vi "test Compile RaF Channel Data.vi"(8 "error in (no error)":errorcluster, 11 "TestCase in":refnum<class "Routing and Faulting Compile Unit Tests.lvclass">) -> (0 "error out":errorcluster, 3 "TestCase out":refnum<class "Routing and Faulting Compile Unit Tests.lvclass">)   [LabVIEW 2020, in "Routing and Faulting Compile Unit Tests.lvclass"]
uses:
  Routing and Faulting Compile Unit Tests.lvclass
  Shared/Channel States.ctl
  Shared/Routing State.ctl
  Shared/Connection.ctl
  Shared/Compiled.Settings.ctl
  Shared/Communication Configuration.ctl
  Shared/Routing and Faulting Configuration.ctl
  Shared/Routing Channel Configuration.ctl
  Shared/Value-Connections Map.ctl
  Shared/Alias Mapping.ctl
  Shared/Alias Endpoint.ctl
  Shared/Compiled Connection.ctl
  Shared/FIFO Indices.ctl
  Routing and Faulting Compile Unit Tests.lvclass/Routing and Faulting Compile Unit Tests.ctl
  System Explorer/Get Channel Data in By Channel ID (offline).vi
  Scripting/Routing and Faulting Scripting.lvlib
  Shared/Routing and Faulting Shared.lvlib
  System Explorer/Routing and Faulting System Explorer.lvlib
panel:
  in  "Save?":bool
  out "Output Filename":string
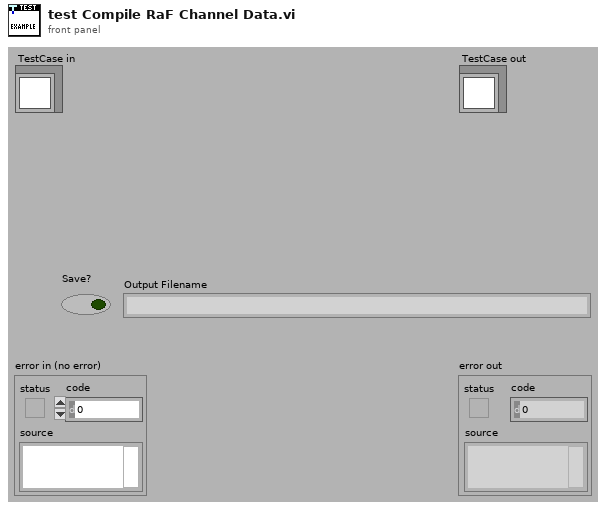
[diagram p1: front panel]
types:
  T1 = typedef "Routing and Faulting Shared.lvlib/Alias Endpoint.ctl" = cluster{"Module Path":string, "Endpoint":string}
  T2 = cluster{"Value-Connections Map.Connection List Array":cluster{"Compiled Connections Indices":i32[]}[]}[]
  T3 = typedef "Routing and Faulting Shared.lvlib/Compiled Connection.ctl" = cluster{"Consumer Queue Index":i32, "Normalized Connection String":string}
  T4 = typedef "Routing and Faulting Shared.lvlib/Communication Configuration.ctl" = cluster{"Consumer Queue Names":string[]}
  T5 = typedef "Routing and Faulting Shared.lvlib/Compiled.Settings.ctl" = cluster{"Custom Device Name":string, "Communication Configuration":T4, "Routing and Faulting Configuration":T6, "Status Channels FIFO Indices":T10}
  T6 = typedef "Routing and Faulting Shared.lvlib/Routing and Faulting Configuration.ctl" = cluster{"Routing Channel Configurations":T7[], "Alias Mappings":T9[], "Compiled Connection Buffer":T3[], "Compiled Initial Connection Indices":i32[]}
  T7 = typedef "Routing and Faulting Shared.lvlib/Routing Channel Configuration.ctl" = cluster{"Channel Name":string, "Initial Value":dbl, "FIFO Index":i32, "Value-Connections Map":T8}
  T8 = typedef "Routing and Faulting Shared.lvlib/Value-Connections Map.ctl" = cluster{"State Value Array":i32[], "Connection List Array":cluster{"Compiled Connections Indices":i32[]}[]}
  T9 = typedef "Routing and Faulting Shared.lvlib/Alias Mapping.ctl" = cluster{"Alias":string, "Endpoint":T1}
  T10 = typedef "Routing and Faulting Shared.lvlib/FIFO Indices.ctl" = cluster{"Status Channel":i32, "Heartbeat Channel":i32}
  T11 = typedef "Routing and Faulting Shared.lvlib/Channel States.ctl" = T12[]
  T12 = typedef "Routing and Faulting Shared.lvlib/Routing State.ctl" = cluster{"Name":string, "Description":string, "Value":i32, "Connection List":T13[]}
  T13 = typedef "Routing and Faulting Shared.lvlib/Connection.ctl" = cluster{"Module":string, "Source":string, "Destination":string}
  T14 = typedef "Custom Device API.lvlib/Custom Device Item Ref.ctl" = u64
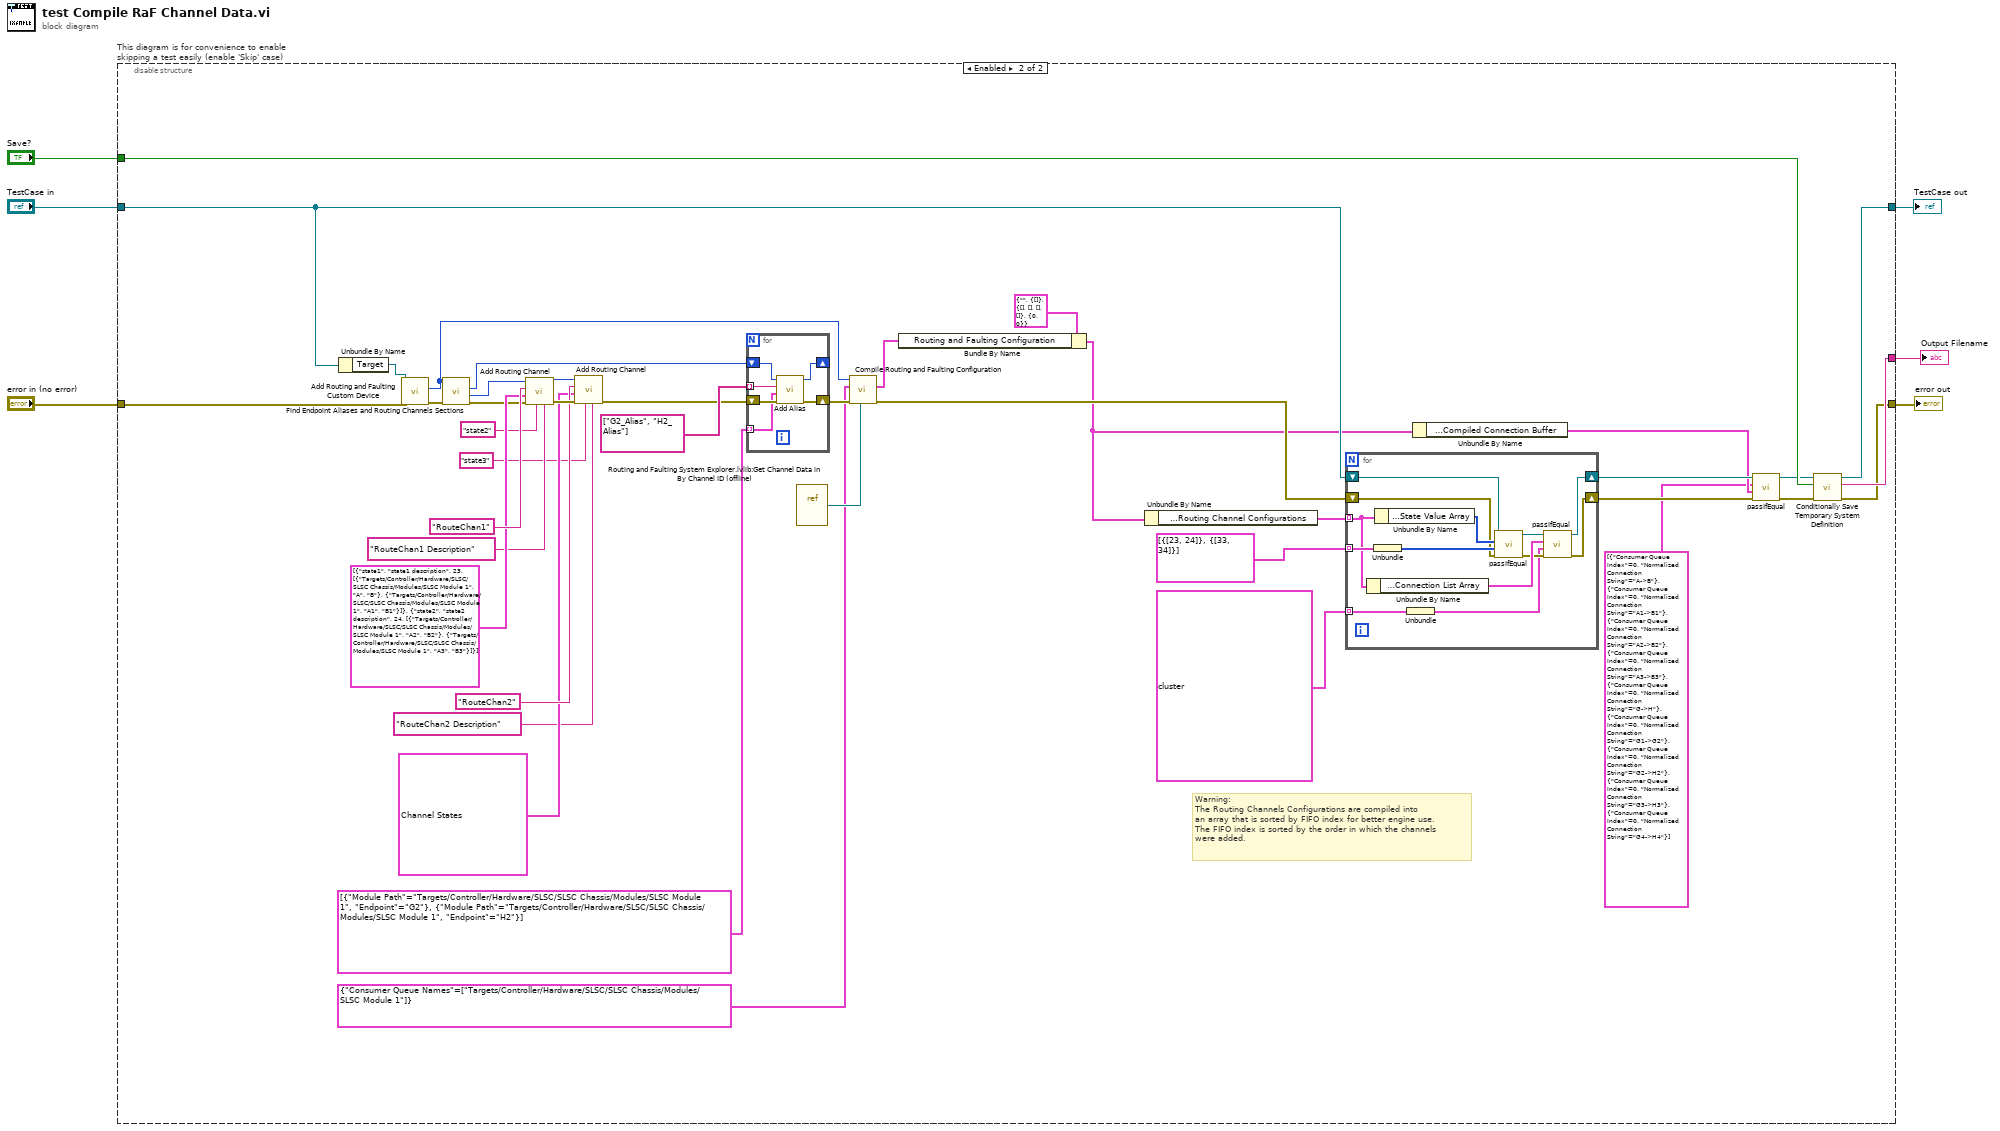
[diagram p0: block diagram]
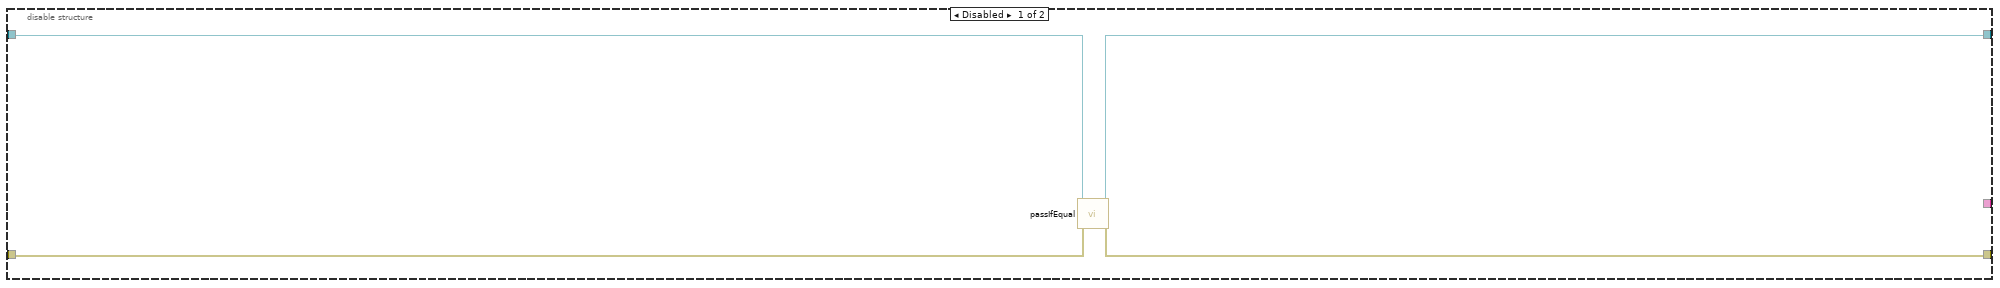
[diagram p2: hidden frame]
diagram:
  n1 = disable-structure "This diagram is for convenience to enable skipping a test easily (enable 'Skip' case)" shown="Enabled" {
    disable-tunnel: "TestCase in" -> [w10 w41]
    disable-tunnel: [w9 w46] -> w3
    disable-tunnel: [w8 w38] -> w5
    disable-tunnel: "error in (no error)" -> [w7 w48]
    disable-tunnel: "Save?" -> [_ w47]
    disable-tunnel: [_ w45] -> w1
    frame Disabled {
      n2 = call-dynamic "passIfEqual.vi"("error in (no error)"=w7, "TestCase in"=w10) -> ("error out"=w8:errorcluster, "TestCase out"=w9:refnum<class "Routing and Faulting Compile Unit Tests.lvclass">)  [unwired: 8 in]
    }
    frame Enabled {
      # "Warning: \nThe Routing Channels Configurations are compiled into\nan array that is sorted by FIFO index for better engine use.\nThe FIFO index is sorted by the order in which the channels\nwere added."
      n3 = Unbundle By Name(w41) -> ("Target"=w49:refnum<k24>)
      n4 = call "Add Routing and Faulting Custom Device.vi"("error in"=w48, "target in"=w49) -> ("error out"=w51:errorcluster, "routing and faulting custom device"=w24:T14)  [unwired: 7 in, 1 out]
      n5 = call "Find Endpoint Aliases and Routing Channels Sections.vi"("error in"=w51, "routing and faulting custom device in"=w24) -> ("error out"=w34:errorcluster, "routing channels"=w33:T14, "endpoint aliases"=w32:T14)  [unwired: 6 in, 1 out]
      n6 = call "Add Routing Channel.vi"("description"="RouteChan1 Description" ("Description"), "initial state"="state2" ("Initial State"), "error in"=w34, "state configurations"=T11 [{"Name"="state1", "Description"="state1 description", "Value"=23, "Connection List"=[{"Module"="Targets/Controller/Hardware/SLSC/SLSC Chassis/Modules/SLSC Module 1", "Source"="A", "Destination"="B"}, {"Module"="Targets/Controller/Hardware/SLSC/SLSC Chassis/Modules/SLSC Module 1", "Source"="A1", "Destination"="B1"}]}, {"Name"="state2", "Description"="state2 description", "Value"=24, "Connection List"=[{"Module"="Targets/Controller/Hardware/SLSC/SLSC Chassis/Modules/SLSC Module 1", "Source"="A2", "Destination"="B2"}, {"Module"="Targets/Controller/Hardware/SLSC/SLSC Chassis/Modules/SLSC Module 1", "Source"="A3", "Destination"="B3"}]}] ("States and Connections"), "channel name"="RouteChan1" ("Channel Name"), "routing channels in"=w33) -> ("error out"=w44:errorcluster, "routing channels out"=w43:T14)  [unwired: 3 in, 1 out]
      n7 = call "Add Routing Channel.vi"("description"="RouteChan2 Description" ("Description"), "initial state"="state3" ("Initial State"), "error in"=w44, "state configurations"=T11 [{"Name"="state3", "Description"="state3 description", "Value"=33, "Connection List"=[{"Module"="Targets/Controller/Hardware/SLSC/SLSC Chassis/Modules/SLSC Module 1", "Source"="G", "Destination"="H"}, {"Module"="Targets/Controller/Hardware/SLSC/SLSC Chassis/Modules/SLSC Module 1", "Source"="G1", "Destination"="G2"}, {"Module"="Targets/Controller/Hardware/SLSC/SLSC Chassis/Modules/SLSC Module 1", "Source"="H2", "Destination"="G2"}]}, {"Name"="state4", "Description"="state4 description", "Value"=34, "Connection List"=[{"Module"="Targets/Controller/Hardware/SLSC/SLSC Chassis/Modules/SLSC Module 1", "Source"="G2", "Destination"="H2"}, {"Module"="Targets/Controller/Hardware/SLSC/SLSC Chassis/Modules/SLSC Module 1", "Source"="G3", "Destination"="H3"}, {"Module"="Targets/Controller/Hardware/SLSC/SLSC Chassis/Modules/SLSC Module 1", "Source"="G4", "Destination"="H4"}]}] ("States and Connections"), "channel name"="RouteChan2" ("Channel Name"), "routing channels in"=w43) -> ("error out"=w36:errorcluster)  [unwired: 3 in, 2 out]
      n8 = for {
        shift-right: [w55] -> _
        shift-left: w32 -> [w56]
        tunnel: string[] ["G2_Alias", "H2_Alias"] -> [w57] mode=indexing
        tunnel: T1[] [{"Module Path"="Targets/Controller/Hardware/SLSC/SLSC Chassis/Modules/SLSC Module 1", "Endpoint"="G2"}, {"Module Path"="Targets/Controller/Hardware/SLSC/SLSC Chassis/Modules/SLSC Module 1", "Endpoint"="H2"}] -> [w52] mode=indexing
        shift-right: [w54] -> w23
        shift-left: w36 -> [w53]
        n9 = call "Add Alias.vi"("error in"=w53, "endpoint"=w52, "alias"=w57, "endpoint aliases in"=w56) -> ("error out"=w54:errorcluster, "endpoint aliases out"=w55:T14)  [unwired: 6 in]
      }
      n10 = vi-ref "Routing and Faulting System Explorer.lvlib:Get Channel Data in By Channel ID (offline).vi"() -> (w22:refnum<vi>)
      n11 = call "Compile Routing and Faulting Configuration.vi"("Get Channel Data Refnum"=w22, "error in (no error)"=w23, "Communication Configuration"=T4 {"Consumer Queue Names"=["Targets/Controller/Hardware/SLSC/SLSC Chassis/Modules/SLSC Module 1"]}, "Device Ref in"=w24) -> ("error out"=w26:errorcluster, "RaF Configuration"=w25:T6)  [unwired: 5 in, 1 out]
      n12 = Bundle By Name(cluster=T5 {"Custom Device Name"="", "Communication Configuration"={"Consumer Queue Names"=[]}, "Routing and Faulting Configuration"={"Routing Channel Configurations"=[], "Alias Mappings"=[], "Compiled Connection Buffer"=[], "Compiled Initial Connection Indices"=[]}, "Status Channels FIFO Indices"={"Status Channel"=0, "Heartbeat Channel"=0}} ("Compiled.Settings.ctl"), "Routing and Faulting Configuration"=w25) -> (w18:T5)
      n13 = Unbundle By Name(w18) -> ("Routing and Faulting Configuration.Routing Channel Configurations"=w19:T7[])
      n14 = for {
        tunnel: w19 -> [w66] mode=indexing
        tunnel: cluster{i32[]}[] [{[23, 24]}, {[33, 34]}] ("expected State Values") -> [w70] mode=indexing
        shift-right: [w63] -> w16
        shift-left: w41 -> [w62]
        shift-right: [w60] -> w17
        shift-left: w26 -> [w61]
        tunnel: T2 [{"Value-Connections Map.Connection List Array"=[{"Compiled Connections Indices"=[0, 1]}, {"Compiled Connections Indices"=[2, 3]}]}, {"Value-Connections Map.Connection List Array"=[{"Compiled Connections Indices"=[4, 5, 6]}, {"Compiled Connections Indices"=[6, 7, 8]}]}] -> [w59] mode=indexing
        n15 = Unbundle By Name(w66) -> ("Value-Connections Map.Connection List Array"=w67:cluster{"Compiled Connections Indices":i32[]}[])
        n16 = Unbundle(w70) -> (w69:i32[])
        n17 = Unbundle By Name(w66) -> ("Value-Connections Map.State Value Array"=w68:i32[])
        n18 = Unbundle(w59) -> ("Value-Connections Map.Connection List Array"=w58:cluster{"Compiled Connections Indices":i32[]}[])
        n19 = call-dynamic "passIfEqual.vi"("error in (no error)"=w61, "y"=w69, "x"=w68, "TestCase in"=w62) -> ("error out"=w65:errorcluster, "TestCase out"=w64:refnum<class "Routing and Faulting Compile Unit Tests.lvclass">)  [unwired: 6 in]
        n20 = call-dynamic "passIfEqual.vi"("error in (no error)"=w65, "y"=w58, "x"=w67, "TestCase in"=w64) -> ("error out"=w60:errorcluster, "TestCase out"=w63:refnum<class "Routing and Faulting Compile Unit Tests.lvclass">)  [unwired: 6 in]
      }
      n21 = Unbundle By Name(w18) -> ("Routing and Faulting Configuration.Compiled Connection Buffer"=w13:T3[])
      n22 = call-dynamic "passIfEqual.vi"("error in (no error)"=w17, "y"=w13, "x"=T3[] [{"Consumer Queue Index"=0, "Normalized Connection String"="A->B"}, {"Consumer Queue Index"=0, "Normalized Connection String"="A1->B1"}, {"Consumer Queue Index"=0, "Normalized Connection String"="A2->B2"}, {"Consumer Queue Index"=0, "Normalized Connection String"="A3->B3"}, {"Consumer Queue Index"=0, "Normalized Connection String"="G->H"}, {"Consumer Queue Index"=0, "Normalized Connection String"="G1->G2"}, {"Consumer Queue Index"=0, "Normalized Connection String"="G2->H2"}, {"Consumer Queue Index"=0, "Normalized Connection String"="G3->H3"}, {"Consumer Queue Index"=0, "Normalized Connection String"="G4->H4"}] ("Routing and Faulting Configuration.Compiled Connection Buffer"), "TestCase in"=w16) -> ("error out"=w14:errorcluster, "TestCase out"=w15:refnum<class "Routing and Faulting Compile Unit Tests.lvclass">)  [unwired: 6 in]
      n23 = call "Conditionally Save Temporary System Definition.vi"("error in (no error)"=w14, "Save?"=w47, "TestCase in"=w15) -> ("error out"=w38:errorcluster, "filename"=w45:string, "TestCase out"=w46:refnum<class "Routing and Faulting Compile Unit Tests.lvclass">)  [unwired: 6 in]
    }
  }
  "error out" <- w5
  "TestCase out" <- w3
  "Output Filename" <- w1
